vi "电流测试.vi"(0 "IT6512C":refnum<visa-resource-name>="GPIB0::16::INSTR", 1 "2700":refnum<visa-resource-name>="GPIB0::16::INSTR", 2 "Ramp Pattern":dbl[](array[numeric]) caption="电流测试点", 5 "error in (no error)":errorcluster) -> (13 "error out":errorcluster, 15 "回读电流":dbl[](array[numeric]), 16 "输入电流":dbl[](array[numeric]), 17 "误差":dbl[](array[numeric]), 18 "斜率":dbl, 19 "截距":dbl)   [LabVIEW 2020]
uses:
  <vilib>/ptbypt/NI_PtbyPt.lvlib
panel:
  in  "Modbus I/O":refnum<visa-resource-name>
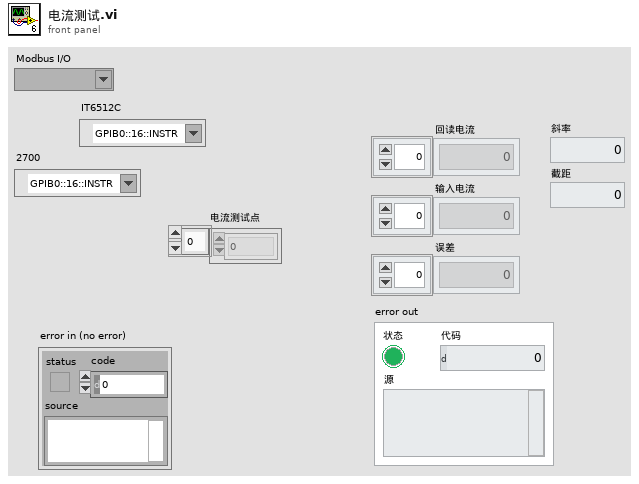
[diagram p1: front panel]
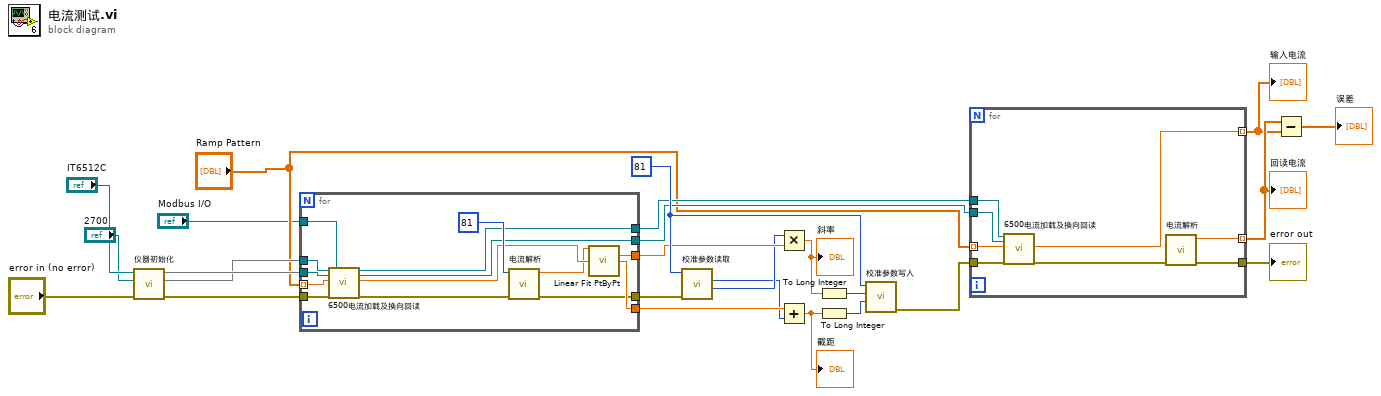
[diagram p0: block diagram]
diagram:
  w20 = u16 81 ("Channel")
  n1 = call "仪器初始化.vi"("错误输入（无错误）"="error in (no error)", 10:"2700", "仪器地址 in"="IT6512C") -> ("error out"=w21:errorcluster, 2:w24, 3:w25)  [unwired: 6 in]
  n2 = for {
    tunnel: "Ramp Pattern" -> [w37] mode=indexing
    tunnel: w25 -> [w39]
    tunnel: w24 -> [w38]
    tunnel: w21 -> [w35]
    tunnel: [w31] -> w19
    tunnel: [w30] -> w16
    tunnel: [w29] -> w13
    tunnel: [w28] -> w9
    tunnel: [w27] -> w8
    tunnel: "Modbus I/O" -> [w26]
    n3 = call "6500电流加载及换向回读.vi"("2700 in"=w38, "IT6512C in"=w39, "输入电流"=w37, "error in"=w35, "Modbus I/O"=w26) -> ("2700 out"=w28:refnum<visa-resource-name>, "IT6512C out"=w27:refnum<visa-resource-name>, "实际电流"=w33:dbl, "error out"=w34:errorcluster)  [unwired: 11 in]
    n4 = call "电流解析.vi"("error in"=w34, "Channel"=u16 81) -> ("error out"=w29:errorcluster, "读取电流"=w32:dbl)  [unwired: 8 in]
    n5 = call <vilib>:"Linear Fit PtByPt.vi"("y"=w32, "x"=w33) -> ("slope"=w31:dbl, "intercept"=w30:dbl)  [unwired: 9 in, 3 out]
  }
  n6 = call "校准参数读取.vi"("error in"=w13, "Channel"=w20) -> ("斜率"=w12:i32, "截距"=w11:i32)  [unwired: 7 in, 1 out]
  n7 = Multiply(x=w12, y=w19) -> (x*y=w18:dbl)
  "斜率" <- w18
  n8 = Add(x=w16, y=w11) -> (x+y=w15:dbl)
  "截距" <- w15
  n9 = To Long Integer(number=w18) -> (32bit integer=w17:i32)
  n10 = To Long Integer(number=w15) -> (32bit integer=w14:i32)
  n11 = call "校准参数写入.vi"("截距"=w14, "斜率"=w17, "Channel"=w20) -> ("error out"=w10:errorcluster)  [unwired: 7 in, 1 out]
  n12 = for {
    tunnel: "Ramp Pattern" -> [w43] mode=indexing
    tunnel: w10 -> [w46]
    tunnel: w9 -> [w45]
    tunnel: w8 -> [w44]
    tunnel: [w42] -> w7 mode=indexing
    tunnel: [w41] -> w6 mode=indexing
    tunnel: [w40] -> w3
    n13 = call "6500电流加载及换向回读.vi"("2700 in"=w45, "IT6512C in"=w44, "输入电流"=w43, "error in"=w46) -> ("实际电流"=w41:dbl, "error out"=w47:errorcluster)  [unwired: 12 in, 2 out]
    n14 = call "电流解析.vi"("error in"=w47) -> ("error out"=w40:errorcluster, "读取电流"=w42:dbl)  [unwired: 9 in]
  }
  "回读电流" <- w7
  "输入电流" <- w6
  "error out" <- w3
  n15 = Subtract(x=w7, y=w6) -> (x-y=→"误差":dbl[])
